vi "Set motion parameters.vi"(7 "path in":path, 8 "error in (no error)":errorcluster, 9 "axis in":u8, 10 "deviceHandle in":u64, 11 "Motion parameters":T1={"Frequency [Hz]"=1000.0, "Precision [m°]"=100.0, "DC voltage [V]"=0.0, "Amplitude [V]"=5.0} {"Amplitude [V]" min=0.1 max=5000.0; "DC voltage [V]" min=1.0 max=1000.0; "Precision [m°]" min=0.0 max=60.0; "Frequency [Hz]" min=0.0 max=60.0}) -> (0 "error out":errorcluster, 1 "Motion parameters out":T1={"Frequency [Hz]"=1000.0, "Precision [m°]"=100.0, "DC voltage [V]"=0.0, "Amplitude [V]"=5.0} {"Amplitude [V]" min=0.1 max=5000.0; "DC voltage [V]" min=1.0 max=1000.0; "Precision [m°]" min=0.0 max=60.0; "Frequency [Hz]" min=0.0 max=60.0}, 2 "axis":u8(ring) items=["1", "2", "3"], 3 "deviceHandle":u64)   [LabVIEW 2024, in "SampleRotator.lvlib"]
doc: "Sets and coerce (if needed) a motion parameters: amplitude[V]; offset voltage [V]; target range[um]; frequency [Hz]\n\ninputs: path; handle; Motion parameters; error cluster\n\noutput: motion parameters, error cluster"
uses:
  SampleRotator.lvlib
  ctl/Motion Properties.ctl
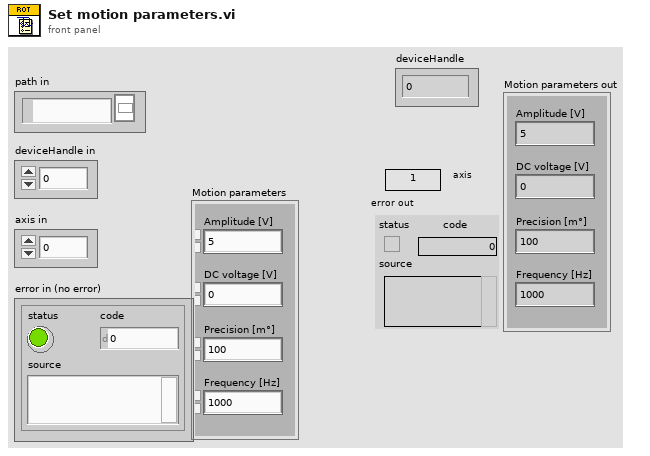
[diagram p1: front panel]
types:
  T1 = typedef "Motion Properties.ctl" = cluster{"Frequency [Hz]":dbl, "Precision [m°]":dbl, "DC voltage [V]":dbl, "Amplitude [V]":dbl}
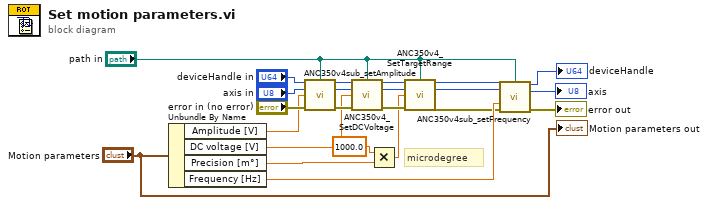
[diagram p0: block diagram]
diagram:
  # "microdegree"
  n1 = Unbundle By Name("Motion parameters") -> ("Amplitude [V]"=w11:dbl, "DC voltage [V]"=w10:dbl, "Precision [m°]"=w9:dbl, "Frequency [Hz]"=w8:dbl)
  n2 = call <instrlib>:"ANC350v4sub_setAmplitude.vi"("deviceHandle"="deviceHandle in", "Path to *.DLL"="path in", "axis"="axis in", "amplitude in"=w11, "error in"="error in (no error)") -> ("deviceHandle"=w14:u64, "axis"=w16:u8, "error ANC350v4_Amplitude"=w19:errorcluster)  [unwired: 8 in]
  n3 = call <instrlib>:"ANC350v4_SetDCVoltage.vi"("deviceHandle"=w14, "Path to *.DLL"="path in", "axis"=w16, "DC voltage"=w10, "error in"=w19) -> ("deviceHandle"=w17:u64, "axis"=w15:u8, "error ANC350v4_setDCVoltage"=w20:errorcluster)  [unwired: 8 in]
  n4 = Multiply(x=1000.0 ("Precision [m°]"), y=w9) -> (x*y=w2:dbl)
  n5 = call <instrlib>:"ANC350v4_SetTargetRange.vi"("deviceHandle"=w17, "Path to *.DLL"="path in", "axis"=w15, "TargetRange [µm | m°]"=w2, "error in"=w20) -> ("deviceHandle"=w5:u64, "axis"=w4:u8, "error ANC350v4_setTargetRange"=w3:errorcluster)  [unwired: 8 in]
  n6 = call <instrlib>:"ANC350v4sub_setFrequency.vi"("deviceHandle"=w5, "Path to *.DLL"="path in", "axis"=w4, "Frequency [Hz] in"=w8, "error in"=w3) -> ("deviceHandle"=→"deviceHandle":u64, "axis"=→"axis":u8, "error ANC350v4_frequency"=→"error out":errorcluster)  [unwired: 8 in]
  "Motion parameters out" <- "Motion parameters"
